vi "Read Refs.vi"(11 "Actor in":refnum<class "Actor.lvclass">) -> (2 "Refs":refnum<class "Refs.lvclass">)   [LabVIEW 2020, in "jettl.lvlib" / "Actor.lvclass"]
uses:
  Actor.lvclass
  Refs/Refs.lvclass
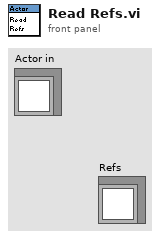
[diagram p1: front panel]
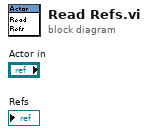
[diagram p0: block diagram]
diagram:
